vi "GetNI_SynthFocus_25_GPU.vi"(0 "Digitizer Settings":T4={"Digitizer delay (us) "=0.0, "rf points per line"=2048, "lines per plane"=128, "Samp Rate (Hz)"=100000000.0, "Additional dig delay (us)"=0.0, "Voltage Scale"=0.4, "Pre-Looks"=0, "Offset delay (us)"=0.0, "bits A/D"=8, "Avg Num"=1, "DigTimeOut"=5.0, "Rel Dig Delay"=0.0, "Dig Ch"=0, "LeCroyCluster"={"LeCroy Channels"=[TRUE, FALSE, FALSE, FALSE], "LC read pt offset"=0.0, "Sweep Avg"=FALSE}, "Main Digitizer"=enum."NI Digitizer", "Dig Config"=enum."Single channel", "Digitizer ID Cluster"={"Acqiris/Alazar/SP ID"=[], "NI Instr Handles"=[], "LeCroy VISA"="", "GaGe Handle"={"Handle"=0, "Sample size"=0, "Resolution"=0, "Offset"=0, "Channels"=0, "Boards"=0}, "ATS Ref"="ATS9350", "Acqiris Address"=["PCI::INSTR0"], "ADQRef"=refnum, "adq_cu_ptr"=refnum}, "Trigger Settings"={"Trig Source"=1, "Trig Coupling"=0, "Trig Slope"=0, "Level (mV)"=1500.0}, "Bulk Acq"=FALSE, "Bulk Start Indexes"=[], "Data Ref RF"=refnum, "NI ID/Channel"=[], "Total Dig CH"=1, "Xtra Ann Trig delay (us)"=10.0, "Fix Z Delay?"=FALSE, "One Way Transmission?"=FALSE, "Data Ref Log"=refnum} {"Trigger Settings"."Trig Slope" items=["Positive", "Negative"]; "Trigger Settings"."Level (mV)" format="%.2f"; "Trigger Settings"."Trig Coupling" items=["DC 1 MOhm", "AC 1 MOhm", "DC 50 Ohm", "AC 50 Ohm"]; "Trigger Settings"."Trig Source" items=["Chan 1", "External"]; "Rel Dig Delay" format="%.2f"; "DigTimeOut" format="%.2f"; "Avg Num" min=1; "Offset delay (us)" format="%.2f"; "Additional dig delay (us)" format="%.2f"; "Digitizer delay (us)" format="%.2f"}, 7 "errorin":errorcluster, 8 "File Array":string[](array[string]), 9 "Ann Array Params":T1={"Synth Foc?"=FALSE, "Focal Zones"=41, "Switch T/R"=0, "Trans Geometry (mm)"={"Transducer"=0, "Geo Focus"=12.0, "a (radius)"=3.0, "# of rings"=5, "kerf space "=0.1, "Center Freq"=12.0}, "Sub Ap Excite?"=FALSE, "Full Array Scan?"=FALSE, "Xmt/Rcv"={"XMIT"=[TRUE, TRUE, TRUE, TRUE, TRUE], "RCV"=[TRUE, TRUE, TRUE, TRUE, TRUE]}, "PulseSpacing (us)"=0.0, "Xmit Ring"=0, "XMIT CHS"=0, "RCV CHS"=0, "GPU?"=FALSE, "Save TIFF?"=FALSE, "downfactor"=1, "RCV 1CH"=0} {"RCV 1CH" items=["All", "1", "2", "3", "4", "5"]; "Trans Geometry (mm)"."Transducer" items=["6D 12R 40 MHz"=0, "10D 31R 20 MHz"=1, "10D 23R 20 MHz"=2, "6D 23R 40 MHz"=3, "4.5D 10.7R 40 MHz"=4, "9D 23.5R 20 MHz"=5, "9D 25.8R 20MHz"=6, "Enter"=99]; "Switch T/R" min=1 max=5 step=1}, 10 "lines per plane":i32, 15 "Reverse?":bool) -> (17 "Raw VGain (scale)":dbl, 18 "Gain Array":T8(array[cluster]), 21 "VGain (dB)":dbl, 27 "error out":errorcluster)   [LabVIEW 2022 SP3]
uses:
  -DigitizerRoutines/DigitizerSettings.ctl
  -DigitizerRoutines/Digitizer.ctl
  -DigitizerRoutines/DigConfig.ctl
  -DigitizerRoutines/DigitizerID.ctl
  C:/Windows/System32/ADQAPI_dotNet_helper.dll
  Windows/System32/ADQAPI_dotNet_helper.dll
  Annular Array/-AnnularRoutines/AnnularArray.ctl
  Annular Array/-AnnularRoutines/TransGeometry.ctl
  Annular Array/-AnnularRoutines/ArrayGeometry.ctl
  <instrlib>/niScope/Acquire/Fetch/niScope Multi Fetch Binary 8.vi
panel:
  out "read time":u32
  out "synth foc time":u32
  out "Numeric":i32
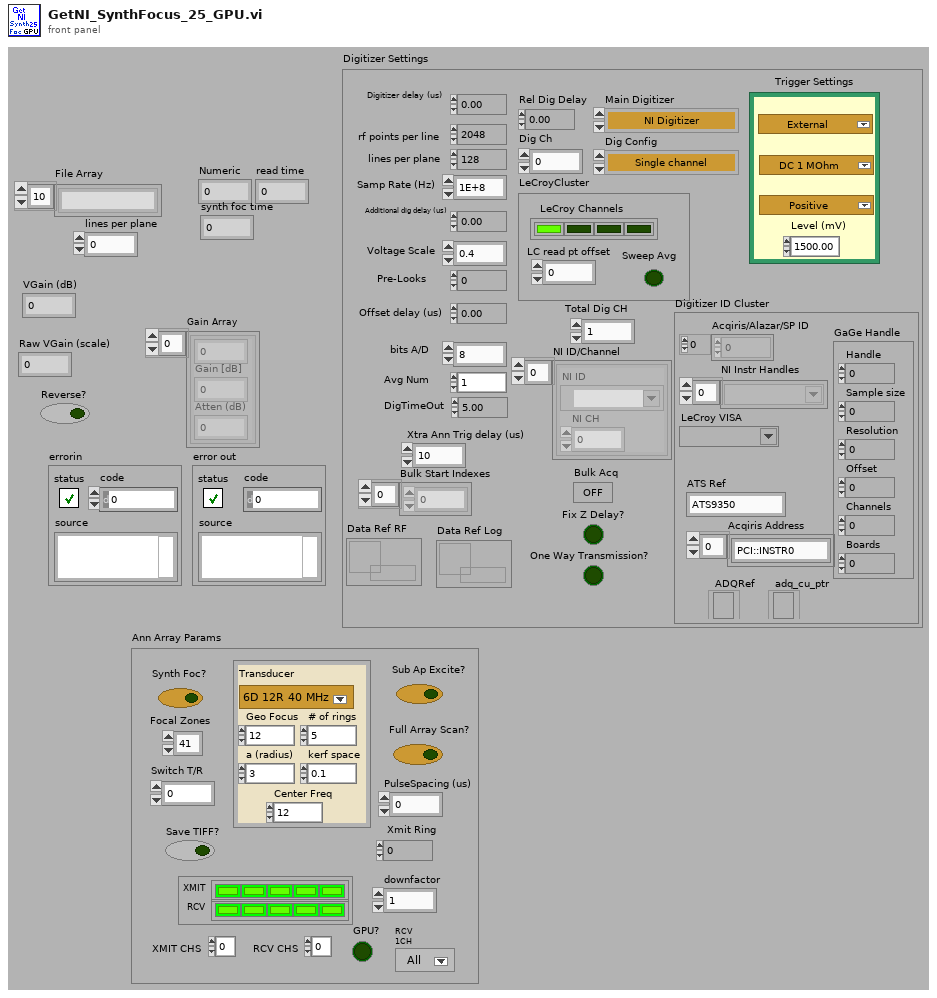
[diagram p1: front panel]
types:
  T1 = typedef "AnnularArray.ctl" = cluster{"Synth Foc?":bool, "Focal Zones":i16, "Switch T/R":i16, "Trans Geometry (mm)":T2, "Sub Ap Excite?":bool, "Full Array Scan?":bool, "Xmt/Rcv":cluster{"XMIT":bool[], "RCV":bool[]}, "PulseSpacing (us)":sgl, "Xmit Ring":i32, "XMIT CHS":u8, "RCV CHS":u8, "GPU?":bool, "Save TIFF?":bool, "downfactor":i32, "RCV 1CH":u16}
  T2 = typedef "TransGeometry.ctl" = cluster{"Transducer":T3, "Geo Focus":dbl, "a (radius)":dbl, "# of rings":i32, "kerf space ":dbl, "Center Freq":dbl}
  T3 = typedef "ArrayGeometry.ctl" = u16
  T4 = typedef "DigitizerSettings.ctl" = cluster{"Digitizer delay (us) ":dbl, "rf points per line":i32, "lines per plane":i32, "Samp Rate (Hz)":dbl, "Additional dig delay (us)":dbl, "Voltage Scale":dbl, "Pre-Looks":i32, "Offset delay (us)":dbl, "bits A/D":i8, "Avg Num":i32, "DigTimeOut":sgl, "Rel Dig Delay":sgl, "Dig Ch":i32, "LeCroyCluster":cluster{"LeCroy Channels":bool[], "LC read pt offset":dbl, "Sweep Avg":bool}, "Main Digitizer":T5, "Dig Config":T6, "Digitizer ID Cluster":T7, "Trigger Settings":cluster{"Trig Source":u16, "Trig Coupling":u16, "Trig Slope":u16, "Level (mV)":dbl}, "Bulk Acq":bool, "Bulk Start Indexes":i32[], "Data Ref RF":refnum<data-value>, "NI ID/Channel":cluster{"NI ID":refnum<k15>, "NI CH":i32}[], "Total Dig CH":i32, "Xtra Ann Trig delay (us)":dbl, "Fix Z Delay?":bool, "One Way Transmission?":bool, "Data Ref Log":refnum<data-value>}
  T5 = typedef "Digitizer.ctl" = enum16{"Acqiris Digitizer", "NI Digitizer", "LeCroy", "GaGe", "AlazarTech", "No Digitizer", "Teledyne"}
  T6 = typedef "DigConfig.ctl" = enum16{"Single channel", "2 Chans w/ 2 Acqiris", "2 Chans w/ 1 Acqiris", "5-CH Pulser New", "5-CH pulser w/ ann array", "5-pass style ann array", "Empty"}
  T7 = typedef "DigitizerID.ctl" = cluster{"Acqiris/Alazar/SP ID":u32[], "NI Instr Handles":refnum<k15>[], "LeCroy VISA":refnum<visa-resource-name>, "GaGe Handle":cluster{"Handle":u32, "Sample size":u32, "Resolution":i32, "Offset":i32, "Channels":u32, "Boards":u32}, "ATS Ref":string, "Acqiris Address":string[], "ADQRef":refnum<k24>, "adq_cu_ptr":refnum<k24>}
  T8 = cluster{sgl, "Gain [dB]  ":sgl, "Atten (dB)":sgl}[]
  T9 = cluster{"actualSamples":i32, "absoluteInitialX":dbl, "relativeInitialX":dbl, "xIncrement":dbl, "offset":dbl, "gain":dbl, "reserved1":dbl, "reserved2":dbl}[]
  T10 = cluster{"actualSamples":i32, "absoluteInitialX":dbl, "relativeInitialX":dbl, "xIncrement":dbl, "offset":dbl, "gain":dbl, "reserved1":dbl, "reserved2":dbl}
  T11 = cluster{sgl, "Gain [dB]  ":sgl, "Atten (dB)":sgl}
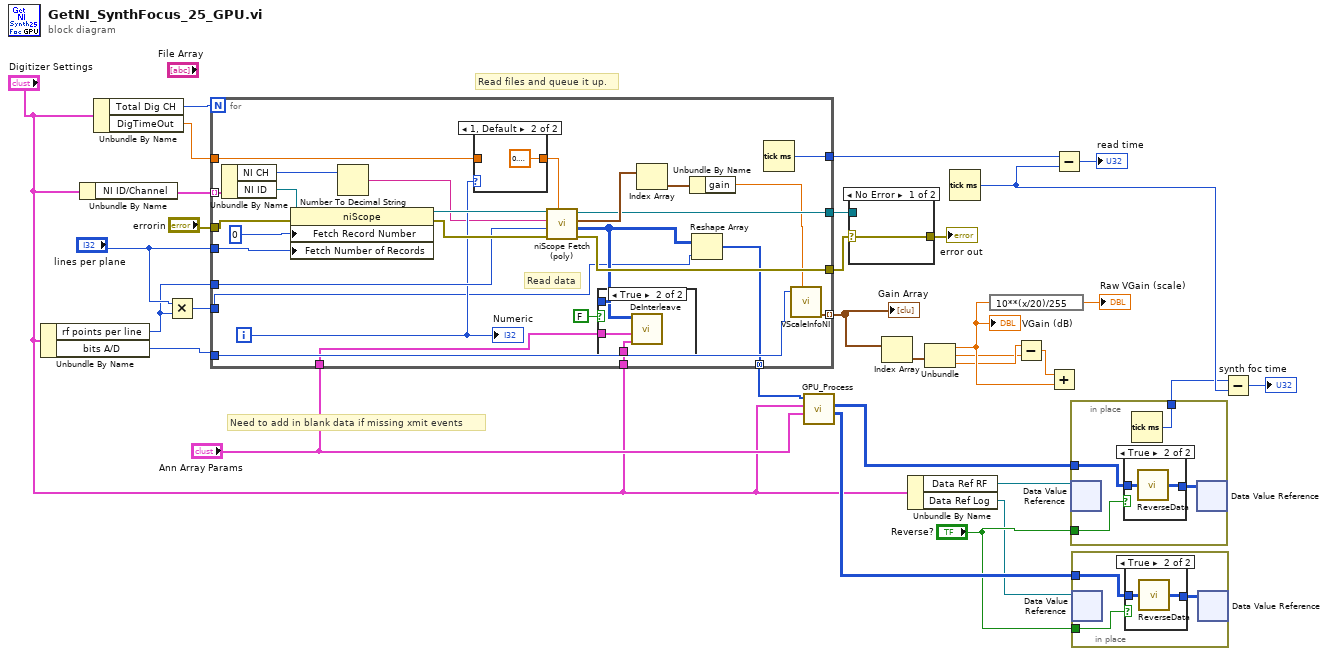
[diagram p0: block diagram]
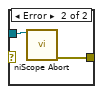
[diagram p4: hidden frame]
diagram:
  # "Need to add in blank data if missing xmit events"
  # "Read files and queue it up."
  n1 = Unbundle By Name("Digitizer Settings") -> ("rf points per line"=w15:i32, "bits A/D"=w14:i8)
  n2 = Unbundle By Name("Digitizer Settings") -> ("NI ID/Channel"=w17:cluster{"NI ID":refnum<k15>, "NI CH":i32}[])
  n3 = Unbundle By Name("Digitizer Settings") -> ("Total Dig CH"=w11:i32, "DigTimeOut"=w7:sgl)
  n4 = Multiply(x="lines per plane", y=w15) -> (x*y=w3:i32)
  n5 = for {
    N: w11 -> [_]
    tunnel: w7 -> [w46]
    tunnel: w15 -> [w50]
    tunnel: "errorin" -> [w58]
    tunnel: "lines per plane" -> [w53]
    tunnel: [w52] -> w29
    tunnel: [w49] -> w22
    tunnel: [w48] -> w21
    tunnel: w17 -> [w44] mode=indexing
    tunnel: w3 -> [w32]
    tunnel: [w34] -> w9 mode=concatenating
    tunnel: w14 -> [w39]
    tunnel: [w38] -> w13 mode=indexing
    tunnel: "Ann Array Params" -> [w36]
    tunnel: "Digitizer Settings" -> [w35]
    i -> [w47]
    # "Read data"
    n6 = Unbundle By Name(w44) -> ("NI CH"=w42:i32, "NI ID"=w43:refnum<k15>)
    n7 = property class="niScope"(reference=w43, error in=w58, "Fetch Record Number"=0, "Fetch Number of Records"=w53) -> (reference out=w51:refnum<k15>, error out=w57:errorcluster)
    n8 = Number To Decimal String(number=w42) -> (decimal integer string=w41:string)  [unwired: 1 in]
    n9 = case shown="1, Default" w47 {
      tunnel: w46 -> [w62 _]
      tunnel: [w62 sgl 0.1 ("DigTimeOut")] -> w45
      frame 0 {
      }
      frame 1, Default {
      }
    }
    n10 = call-poly <instrlib>:"niScope Fetch (poly).vi"("timeout"=w45, "error in"=w57, "numSamples"=w50, "channels"=w41, "instrument handle"=w51) -> ("error out"=w49:errorcluster, "wfm"=w37:i8[][], "wfm info"=w56:T9, "instrument handle out"=w52:refnum<k15>)  [unwired: 3 out]
    n11 = case shown="True" FALSE {
      tunnel: w37 -> [_ w61]
      tunnel: w36 -> [_ w60]
      tunnel: w35 -> [_ w59]
      frame False {
      }
      frame True {
        n12 = call "DeInterleave.vi"("Digitizer Settings"=w59, "Ann Array Params"=w60, "Data in"=w61) -> ()  [unwired: 8 in, 1 out]
      }
    }
    n13 = Index Array(array=w56) -> (element=w55:T10)  [unwired: 1 in]
    n14 = Unbundle By Name(w55) -> ("gain"=w40:dbl)
    n15 = Reshape Array(w37, w32) -> (w34:i8[])
    n16 = Tick Count (ms)() -> (millisecond timer value=w48:u32)
    n17 = call "VScaleInfoNI.vi"("A/D bits"=w39, "gain"=w40) -> ("Voltage Scale"=w38:T11)  [unwired: 5 in, 3 out]
    "Numeric" <- w47
  }
  "Gain Array" <- w13
  n18 = call "GPU_Process.vi"("Ann Array Params"="Ann Array Params", "Digitizer Settings"="Digitizer Settings", "Raw Data In"=w9) -> ("RFimageData"=w6:i16[][], "RF_Out"=w8:i16[][])  [unwired: 6 in, 1 out]
  n19 = case shown="No Error" w22 {
    selector: w22 -> [w64 _]
    tunnel: w29 -> [_ w66]
    tunnel: [w64 w65] -> w30
    frame No Error {
    }
    frame Error {
      n20 = call <instrlib>:"niScope Abort.vi"("instrument handle"=w66) -> ("error out"=w65:errorcluster)  [unwired: 1 in, 13 out]
    }
  }
  "error out" <- w30
  n21 = Index Array(array=w13) -> (element=w28:T11)  [unwired: 1 in]
  n22 = Unbundle By Name("Digitizer Settings") -> ("Data Ref RF"=w12:refnum<data-value>, "Data Ref Log"=w4:refnum<data-value>)
  n23 = Unbundle(w28) -> (w27:sgl, "Gain [dB]"=w25:sgl, "Atten (dB)"=w26:sgl)
  "VGain (dB)" <- w27
  n24 = Tick Count (ms)() -> (millisecond timer value=w20:u32)
  n25 = expression code="10**(x/20)/255"(w27) -> (→"Raw VGain (scale)":sgl)
  n26 = Subtract(x=w26, y=w25) -> (x-y=w24:sgl)
  n27 = Add(x=w24, y=w27) -> ()  [unwired: 1 out]
  n28 = Subtract(x=w21, y=w20) -> (x-y=→"read time":u32)
  n29 = in-place {
    in-place-border: w8 -> [w68]
    in-place-border: [w70] -> w10
    in-place-border: "Reverse?" -> [w67]
    n30 = in-place-dvr #1(w12) -> ()  [unwired: 2 out]
    n31 = case shown="True" w67 {
      tunnel: w68 -> [w71 w73]
      tunnel: [w71 w72] -> w69
      frame False {
      }
      frame True {
        n32 = call "ReverseData.vi"("Array in"=w73) -> ("Array out"=w72:i16[][])
      }
    }
    n33 = Tick Count (ms)() -> (millisecond timer value=w70:u32)
    n34 = in-place-dvr #1(w69) -> ()  [unwired: 2 out]
  }
  n35 = in-place {
    in-place-border: w6 -> [w75]
    in-place-border: "Reverse?" -> [w74]
    n36 = in-place-dvr #2(w4) -> ()  [unwired: 2 out]
    n37 = case shown="True" w74 {
      tunnel: w75 -> [w77 w79]
      tunnel: [w77 w78] -> w76
      frame False {
      }
      frame True {
        n38 = call "ReverseData.vi"("Array in"=w79) -> ("Array out"=w78:i16[][])
      }
    }
    n39 = in-place-dvr #2(w76) -> ()  [unwired: 2 out]
  }
  n40 = Subtract(x=w10, y=w20) -> (x-y=→"synth foc time":u32)
